vi "if_v0_v3.vi"() -> ()   [LabVIEW 2010]
panel:
  in  "Selectie":bool
  in  "Numeric 2":u8=170
  in  "Numeric":u8=85
  out "Array":bool[](array[boolean])=[TRUE, FALSE, TRUE, FALSE, TRUE, FALSE, TRUE, FALSE]
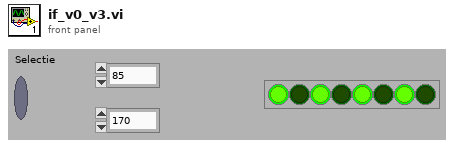
[diagram p1: front panel]
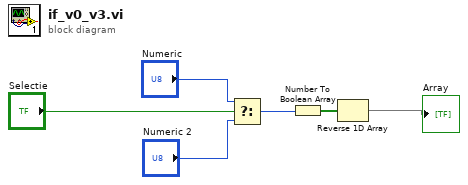
[diagram p0: block diagram]
diagram:
  n1 = Select(t="Numeric", s="Selectie", f="Numeric 2") -> (s? t:f=w1:u8)
  n2 = Number To Boolean Array(number=w1) -> (Boolean array=w6:bool[])
  n3 = Reverse 1D Array(array=w6) -> (reversed array=→"Array":bool[])
